vi "FIR_4decimate_5cycles_32bit.vi"(7 "reset":bool, 8 "valid in":bool, 10 "Q in":fxp<+/-,32,14>, 11 "I in":fxp<+/-,32,14>) -> (0 "valid out":bool, 2 "Q out":fxp<+/-,32,14>, 3 "I out":fxp<+/-,32,14>, 4 "ready for input":bool)   [LabVIEW 2025]
uses:
  <vilib>/rvi/IPIntegrationNode/IPINode_Typedef/niFpgaIPINodeSupportedFamilies.ctl
  <vilib>/rvi/FXPMathLib/FxpConvert/subVIs/nifxpmath_Convert_SimConfig.ctl
  <vilib>/fxp/LVFixedPointQuantizationPolicyTypeDef.ctl
  <vilib>/fxp/LVFixedPointOverflowPolicyTypeDef.ctl
  <vilib>/rvi/IPIntegrationNode/IPINode_Utilities/niFpgaIPINodeSimCore.vi
  <vilib>/rvi/FXPMathLib/FxpConvert/simVIs/DllFxpConvertTemp_sub.vi
  <vilib>/rvi/XilinxIP/XIPIN_XNode/niFpgaXIPIN.xnode
  Xilinx/FIR_4decimate_5cycles_32bit/xsim.dir/FIR_4decimate_5cycles_32bit_E47772A9C93441649D63D6FCF55627B3/xsimk_E47772A9C93441649D63D6FCF55627B3.dll
  <vilib>/rvi/IPIntegrationNode/IPINode_Xnode/niFpgaIPINode.xnode
  <vilib>/rvi/FXPMathLib/FxpInterpret/XNode/nifxpmath_Interpret.xnode
  <vilib>/rvi/FXPMathLib/FxpConvert/XNode/nifxpmath_Convert.xnode
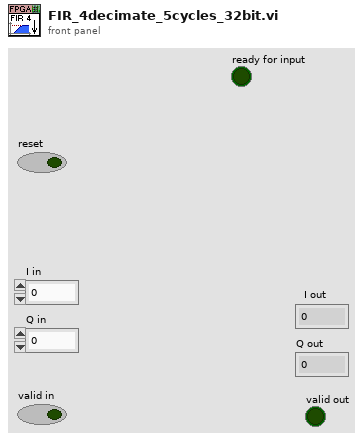
[diagram p1: front panel]
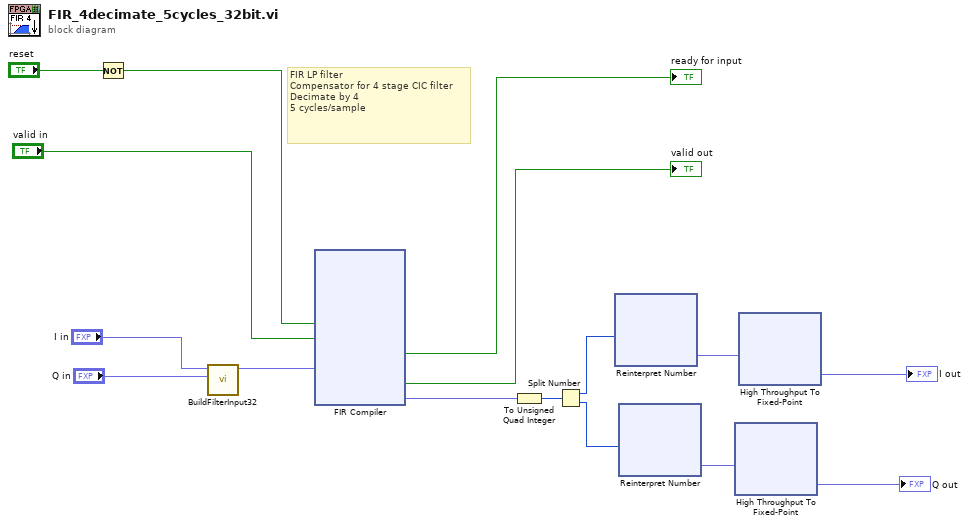
[diagram p0: block diagram]
diagram:
  # "FIR LP filter\nCompensator for 4 stage CIC filter\nDecimate by 4\n5 cycles/sample"
  n1 = Not(x="reset") -> (.not. x?=w6:bool)
  n2 = call "BuildFilterInput32.vi"("Q in"="Q in", "I in"="I in") -> ("Filter input"=w4:fxp<+,64,64>)  [unwired: 9 in]
  n3 = xnode ("FIR Compiler")("aresetn"=w6, "s_axis_data_tvalid"="valid in", "s_axis_data_tdata"=w4) -> ("s_axis_data_tready"=→"ready for input":bool, "m_axis_data_tvalid"=→"valid out":bool, "m_axis_data_tdata"=w1:fxp<+,64,64>)  [unwired: 1 in]
  n4 = To Unsigned Quad Integer(1:w1) -> (0:w12:u64)
  n5 = Split Number(x=w12) -> (hi(x)=w13:u32, lo(x)=w9:u32)
  n6 = xnode "Reinterpret Number"("x"=w13) -> ("y"=w10:fxp<+/-,32,16>)
  n7 = xnode "Reinterpret Number"("x"=w9) -> ("y"=w11:fxp<+/-,32,16>)
  n8 = xnode "High Throughput To Fixed-Point"("x"=w11) -> ("y"=→"Q out":fxp<+/-,32,14>)
  n9 = xnode "High Throughput To Fixed-Point"("x"=w10) -> ("y"=→"I out":fxp<+/-,32,14>)
